vi "Execute.vi"(6 "Index [-1]":i32=-1, 7 "Composite Object":refnum<class "CConfig Object.lvclass">, 8 "error in (no error)":errorcluster, 9 "Results":string[][](array[string]), 11 "Config Query in":refnum<class "Set Query.lvclass">) -> (0 "error out":errorcluster, 1 "Results":string[][](array[string]), 2 "Result":bool, 3 "Config Query out":refnum<class "Set Query.lvclass">, 4 "Index":i32, 5 "Composite Object":refnum<class "CConfig Object.lvclass">)   [LabVIEW 2013, in "Set Query.lvclass"]
doc: "Copyright 2018, Carya Automatisering, Wiebe Walstra."
uses:
  Set Query.lvclass
  CConfig Object.lvclass
  Set Query.lvclass/Set Query.ctl
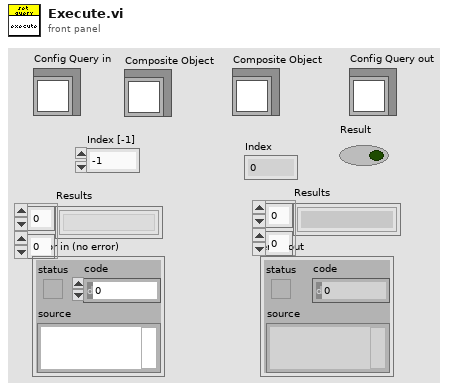
[diagram p1: front panel]
types:
  T1 = typedef "CConfig Object.lvclass/Data.ctl" = enum16{"pre", "name", "middle", "value", "post", "newline", "persistant", "tagged", "type"}
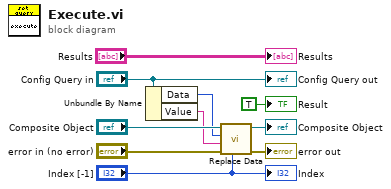
[diagram p0: block diagram]
diagram:
  n1 = Unbundle By Name("Config Query in") -> ("Data"=w2:T1, "Value"=w1:string)
  n2 = call-dynamic "Replace Data.vi"("Index in"="Index [-1]", "error in (no error)"="error in (no error)", "Value"=w1, "Data"=w2, "Composite Object in"="Composite Object") -> ("error out"=→"error out":errorcluster, "Composite Object out"=→"Composite Object":refnum<class "CConfig Object.lvclass">)  [unwired: 5 in]
  "Config Query out" <- "Config Query in"
  "Result" <- TRUE ("Result")
  "Index" <- "Index [-1]"
  "Results" <- "Results"
